vi "DutyM1M2.vi"() -> ()   [LabVIEW 2015, in "Ion Motion Roboclaw.lvlib"]
uses:
  <instrlib>/Ion Motion Roboclaw/Ion Motion Roboclaw.lvlib
panel:
  out "VISA Refnum out":refnum<visa-resource-name>
  out "Valid":bool
  out "error out":errorcluster
  in  "VISA Refnum in":refnum<visa-resource-name>
  in  "Address":u8
  in  "error in (no error)":errorcluster
  in  "Arg1":u16 max=127 step=1
  in  "Arg2":u16 max=127 step=1
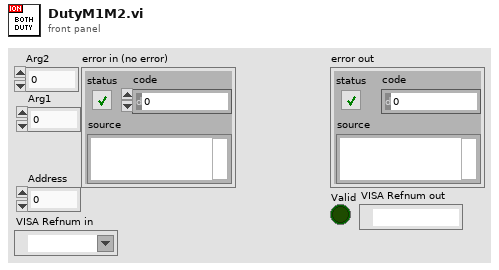
[diagram p1: front panel]
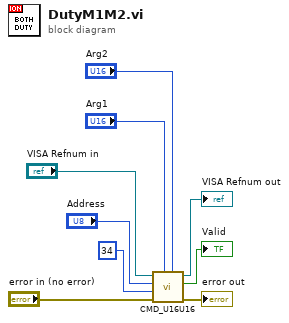
[diagram p0: block diagram]
diagram:
  n1 = call <instrlib>:"CMD_U16U16.vi"("Arg2"="Arg2", "Arg1"="Arg1", "error in (no error)"="error in (no error)", "Cmd"=u8 34, "Address"="Address", "VISA Refnum in"="VISA Refnum in") -> ("error out"=→"error out":errorcluster, "Valid"=→"Valid":bool, "VISA Refnum out"=→"VISA Refnum out":refnum<visa-resource-name>)  [unwired: 3 in]
